vi "Write Values on Buttons.vi"(10 "Coin Array":string[](array[string]), 11 "appended array":refnum<vi>[](array[refnum])) -> ()   [LabVIEW 2020]
doc: "Sets the boolean text of each button acording to .ini file."
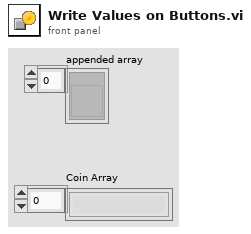
[diagram p1: front panel]
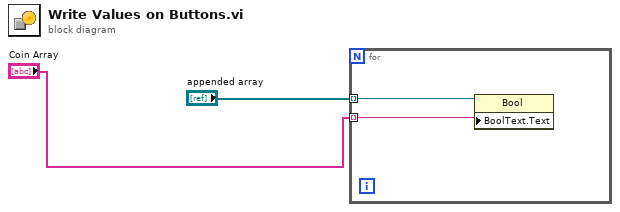
[diagram p0: block diagram]
diagram:
  n1 = for {
    tunnel: "appended array" -> [w4] mode=indexing
    tunnel: "Coin Array" -> [w3] mode=indexing
    n2 = property class="Bool"(reference=w4, "BoolText.Text"=w3) -> ()  [unwired: 1 in, 2 out]
  }
